vi "Begin.vi"(8 "error in":errorcluster) -> (0 "error out":errorcluster)   [LabVIEW 2018]
doc: "Called before other user functions, this VI is expected to open initial I/O refnums, load in file data, and do all program initialization. Notice that the <B>error out</B> terminal is simply used for data flow. Wiring it to other structures or subVIs ensures that this VI runs first."
uses:
  <vilib>/Rock Robotics/WPI/Encoder/WPI_EncoderType.ctl
  <vilib>/Rock Robotics/WPI/DriverStation/WPI_DriverStationRobotMode2.ctl
  <vilib>/Rock Robotics/WPI/Joystick/WPI_JoystickDeviceEnum.ctl
  <vilib>/Rock Robotics/SystemInterfaces/spilib/spi_bus.ctl
  <vilib>/Rock Robotics/WPI/Solenoid/WPI_SolenoidChannel.ctl
  <vilib>/Rock Robotics/SystemInterfaces/DIO/FPGA_DIOPWMChannel.ctl
  <vilib>/Rock Robotics/SystemInterfaces/DIO/FPGA_DIOChannel.ctl
  Robot Global Data.vi
  <vilib>/Rock Robotics/WPI/MotorControl/WPI_MotorControlOpen VictorSP.vi
  <vilib>/Rock Robotics/WPI/Counter/WPI_CounterDigitalInputToDigitalSource.vi
  <vilib>/Rock Robotics/WPI/Solenoid/WPI_SolenoidOpenDouble.vi
  navX-MXP Library/navX-MXP IMU.lvlib
  navX-MXP Library/SERIAL/IO/NI WPI/WPI_SerialPort_USB.ctl
  <vilib>/Rock Robotics/WPI/CAN/TalonSRX/WPI_CANTalonSRX_APIFeedbackSelect.ctl
  <vilib>/Rock Robotics/WPI/CAN/TalonSRX/WPI_CANTalonSRX_APIControlMode.ctl
  <vilib>/Rock Robotics/WPI/MotorControl/WPI_MotorControlOpen SD540.vi
  <vilib>/Rock Robotics/WPI/Gyro/WPI_GyroAnalogOpen.vi
panel:
  in  "Invert Direction":bool
  in  "Decoding Type":T1=enum."4x"
  in  "DistancePerCount":dbl=0.0184
  # "comp:\n?\nprac:\n0.026"
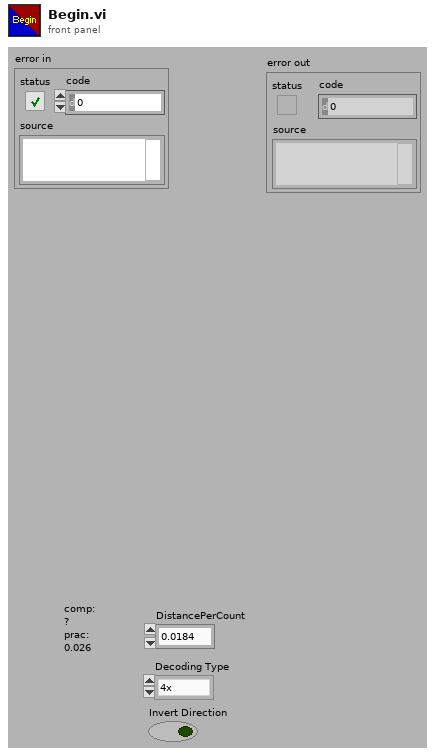
[diagram p1: front panel]
types:
  T1 = typedef "WPI_EncoderType.ctl" = enum16{"1x", "2x", "4x"}
  T2 = typedef "FPGA_DIOChannel.ctl" = enum8{"DIO 0", "DIO 1", "DIO 2", "DIO 3", "DIO 4", "DIO 5", "DIO 6", "DIO 7", "DIO 8", "DIO 9", "DIO MXP 0", "DIO MXP 1", "DIO MXP 2", "DIO MXP 3", "DIO MXP 4", "DIO MXP 5", "DIO MXP 6", "DIO MXP 7", "DIO MXP 8", "DIO MXP 9", "DIO MXP 10", "DIO MXP 11", "DIO MXP 12", "DIO MXP 13", "DIO MXP 14", "DIO MXP 15", "SPI Port CS1", "SPI Port CS2", "SPI Port CS3", "SPI Port MISO", "SPI Port MOSI", "Invalid"}
  T3 = typedef "FPGA_DIOPWMChannel.ctl" = enum8{"PWM 0", "PWM 1", "PWM 2", "PWM 3", "PWM 4", "PWM 5", "PWM 6", "PWM 7", "PWM 8", "PWM 9", "PWM MXP 0", "PWM MXP 1", "PWM MXP 2", "PWM MXP 3", "PWM MXP 4", "PWM MXP 5", "PWM MXP 6", "PWM MXP 7", "PWM MXP 8", "PWM MXP 9", "Invalid"}
  T4 = typedef "WPI_SolenoidChannel.ctl" = enum8{"Solenoid 0", "Solenoid 1", "Solenoid 2", "Solenoid 3", "Solenoid 4", "Solenoid 5", "Solenoid 6", "Solenoid 7", "Invalid"}
  T5 = typedef "spi_bus.ctl" = enum16{"SPI On-Board, CS0", "SPI On-Board, CS1", "SPI On-Board, CS2", "SPI On-Board, CS3", "SPI MXP", "Invalid"}
  T6 = typedef "WPI_JoystickDeviceEnum.ctl" = enum16{"USB 0", "USB 1", "USB 2", "USB 3", "USB 4", "USB 5"}
  T7 = typedef "WPI_DriverStationRobotMode2.ctl" = enum16{"Autonomous Disabled", "Autonomous Enabled", "Teleop Disabled", "Teleop Enabled", "Disconnected", "Finish", "Test Disabled", "Test Enabled", "Emergency Stopped"}
  T8 = typedef "WPI_DigitalInputDevRef.ctl" = cluster{"DevStatus":errorcluster, "DIO Channel":T2}
  T9 = typedef "FPGA_CounterEncoderSourceConvertionLVSourceType.ctl" = cluster{"DevStatus":errorcluster, "AnalogTriggerMode?":bool, "DigitalMode":cluster{"DIO Channel":T10}, "AnalogTriggerMode":cluster{"AnalogTriggerIndex":T11, "OutputType":T12}}
  T10 = typedef "FPGA_DIODigitalSourceChannel.ctl" = enum8{"DIO 0", "DIO 1", "DIO 2", "DIO 3", "DIO 4", "DIO 5", "DIO 6", "DIO 7", "DIO 8", "DIO 9", "DIO MXP 0", "DIO MXP 1", "DIO MXP 2", "DIO MXP 3", "DIO MXP 4", "DIO MXP 5", "DIO MXP 6", "DIO MXP 7", "DIO MXP 8", "DIO MXP 9", "DIO MXP 10", "DIO MXP 11", "DIO MXP 12", "DIO MXP 13", "DIO MXP 14", "DIO MXP 15", "SPI Port CS1", "SPI Port CS2", "SPI Port CS3", "SPI Port MISO", "SPI Port MOSI", "Disabled"}
  T11 = typedef "FPGA_AnalogTriggerIndex.ctl" = enum8{"Trig 0", "Trig 1", "Trig 2", "Trig 3", "Trig 4", "Trig 5", "Trig 6", "Trig 7", "Invalid"}
  T12 = typedef "FPGA_AnalogTriggerOutType.ctl" = enum16{"InWindow", "TriggerState", "Rising", "Falling"}
  T13 = typedef "WPI_EncoderDevRef.ctl" = cluster{"DevStatus":errorcluster, "EncoderIndex":T14, "CounterIndex":T15, "DistancePerCount":dbl, "Decoding Type":T1}
  T14 = typedef "FPGA_EncoderIdx.ctl" = enum8{"Enc 0", "Enc 1", "Enc 2", "Enc 3", "Enc 4", "Enc 5", "Enc 6", "Enc 7", "Invalid"}
  T15 = typedef "FPGA_CounterCtrSystemIndex.ctl" = enum8{"Ctr 0", "Ctr 1", "Ctr 2", "Ctr 3", "Ctr 4", "Ctr 5", "Ctr 6", "Ctr 7", "Invalid"}
  T16 = typedef "WPI_GyroDevRef.ctl" = cluster{"DevStatus":errorcluster, "Analog Channel":T17, "Gain (VoltsPerDegree/Second)":dbl, "Gyro Type":enum16{"Analog", "XRS450"}, "Handle":i32, "SPI Bus":T5, "Device Found":bool, "Sample Rate":dbl, "Calibrate On Open":bool, "Offset":dbl}
  T17 = typedef "FPGA_AIChannel.ctl" = enum8{"AI 0", "AI 1", "AI 2", "AI 3", "AI MXP 0", "AI MXP 1", "AI MXP 2", "AI MXP 3", "Invalid"}
  T18 = typedef "WPI_MotorControlDeviceRef.ctl" = cluster{"DeviceStatus":errorcluster, "Type":T19, "PWM":cluster{"PWM Channel":T3, "DeadBand":T20}, "CAN":cluster{"Device Number":u8, "SetOutput VI Ref":variant, "GetOutput VI Ref":variant, "Enable VI Ref":variant, "Disable VI Ref":variant, "Data":variant}, "Invert":bool, "DIO PWM":cluster{"PWM \"Enable\" Channel":T3, "DIOChannel":T2, "PWM Rate":dbl}}
  T19 = typedef "WPI_MotorControlType.ctl" = enum16{"PWM", "CAN", "DIO PWM"}
  T20 = typedef "WPI_PWMDeadband.ctl" = cluster{"Name":string, "maxPositivePwm":i32, "minPositivePwm":i32, "centerPwm":i32, "maxNegativePwm":i32, "minNegativePwm":i32, "angularRange":u16}
  T21 = typedef "WPI_SolenoidDevRef.ctl" = cluster{"DevStatus":errorcluster, "Pneumatics Control Module":u8, "Forward Solenoid Channel":T4, "Reverse Solenoid Channel":T4}
  T22 = typedef "navX-MXP IMU.lvlib/navX SPI DevRef.ctl" = cluster{"SPIDevRef":T23, "Board Information":T24, "Status":T25, "Offsets":cluster{"Yaw":dbl, "Quat W":dbl, "Quat X":dbl, "Quat Y":dbl, "Quat Z":dbl}, "Update Rate (4Hz-60Hz)":u8, "refnum name":string, "error":errorcluster}
  T23 = typedef "WPI_SPIDevRef.ctl" = cluster{"DevStatus":errorcluster, "Handle":i32, "SPI Bus":T5}
  T24 = typedef "navX-MXP IMU.lvlib/navX Board Information.ctl" = cluster{"WhoAmI (50 | 0x32)":u8, "Board Revision":u8, "Firmware Major Version":u8, "Firmware Minor Version":u8}
  T25 = typedef "navX-MXP IMU.lvlib/navX Status Data.ctl" = cluster{"Update Rate Hz":u8, "Accelerometer Full-Scale Range":u8, "Gyro Full-Scale Range":u16, "NAVX_OP_STATUS":T26, "NAVX_CAL_STATUS":T27, "NAVX_SELFTEST_STATUS":u8, "NAVX_SENSOR_STATUS":T28}
  T26 = typedef "navX-MXP IMU.lvlib/navX NAVX_OP_STATUS.ctl" = u8
  T27 = typedef "navX-MXP IMU.lvlib/navX NAVX_CAL_STATUS.ctl" = u8
  T28 = typedef "navX-MXP IMU.lvlib/navX NAVX_SENSOR_STATUS.ctl" = cluster{"MOVING":bool, "YAW_STABLE":bool, "MAG_DISTURBANCE":bool, "ALTITUDE_VALID":bool, "SEALEVEL_PRESS_SET":bool, "FUSED_HEADING_VALID":bool}
  T29 = typedef "WPI_JoystickDevRef.ctl" = cluster{"Device":T6}
  T30 = typedef "WPI_CANTalonSRX_APIControlMode.ctl" = enum8{"Percent VBus", "Speed", "Position", "Slave", "Unchanged / Invalid"}
  T31 = typedef "WPI_CANTalonSRX_APIFeedbackSelect.ctl" = enum16{"Digital Quadrature Encoder", "Analog Potentiometer", "Analog Encoder"}
  T32 = typedef "navX-MXP IMU.lvlib/WPI_SerialPort_USB.ctl" = enum16{"Onboard RS-232", "MXP TTL", "USB"}
  T33 = typedef "navX-MXP IMU.lvlib/navX Serial DevRef.ctl" = cluster{"SerialPortRef":T34, "Board Information":T24, "Status":T25, "Offsets":cluster{"Yaw":dbl, "Quat W":dbl, "Quat X":dbl, "Quat Y":dbl, "Quat Z":dbl}, "Update Rate (4Hz-60Hz)":u8, "Nav6Mode (YPR)":T35, "refnum name":string, "error":errorcluster}
  T34 = typedef "WPI_SerialPortRef.ctl" = cluster{"DevStatus":errorcluster, "Serial Port Name":refnum<visa-resource-name>}
  T35 = typedef "navX-MXP IMU.lvlib/navX Serial Mode.ctl" = enum16{"YPR", "Gyro", "Quaternion"}
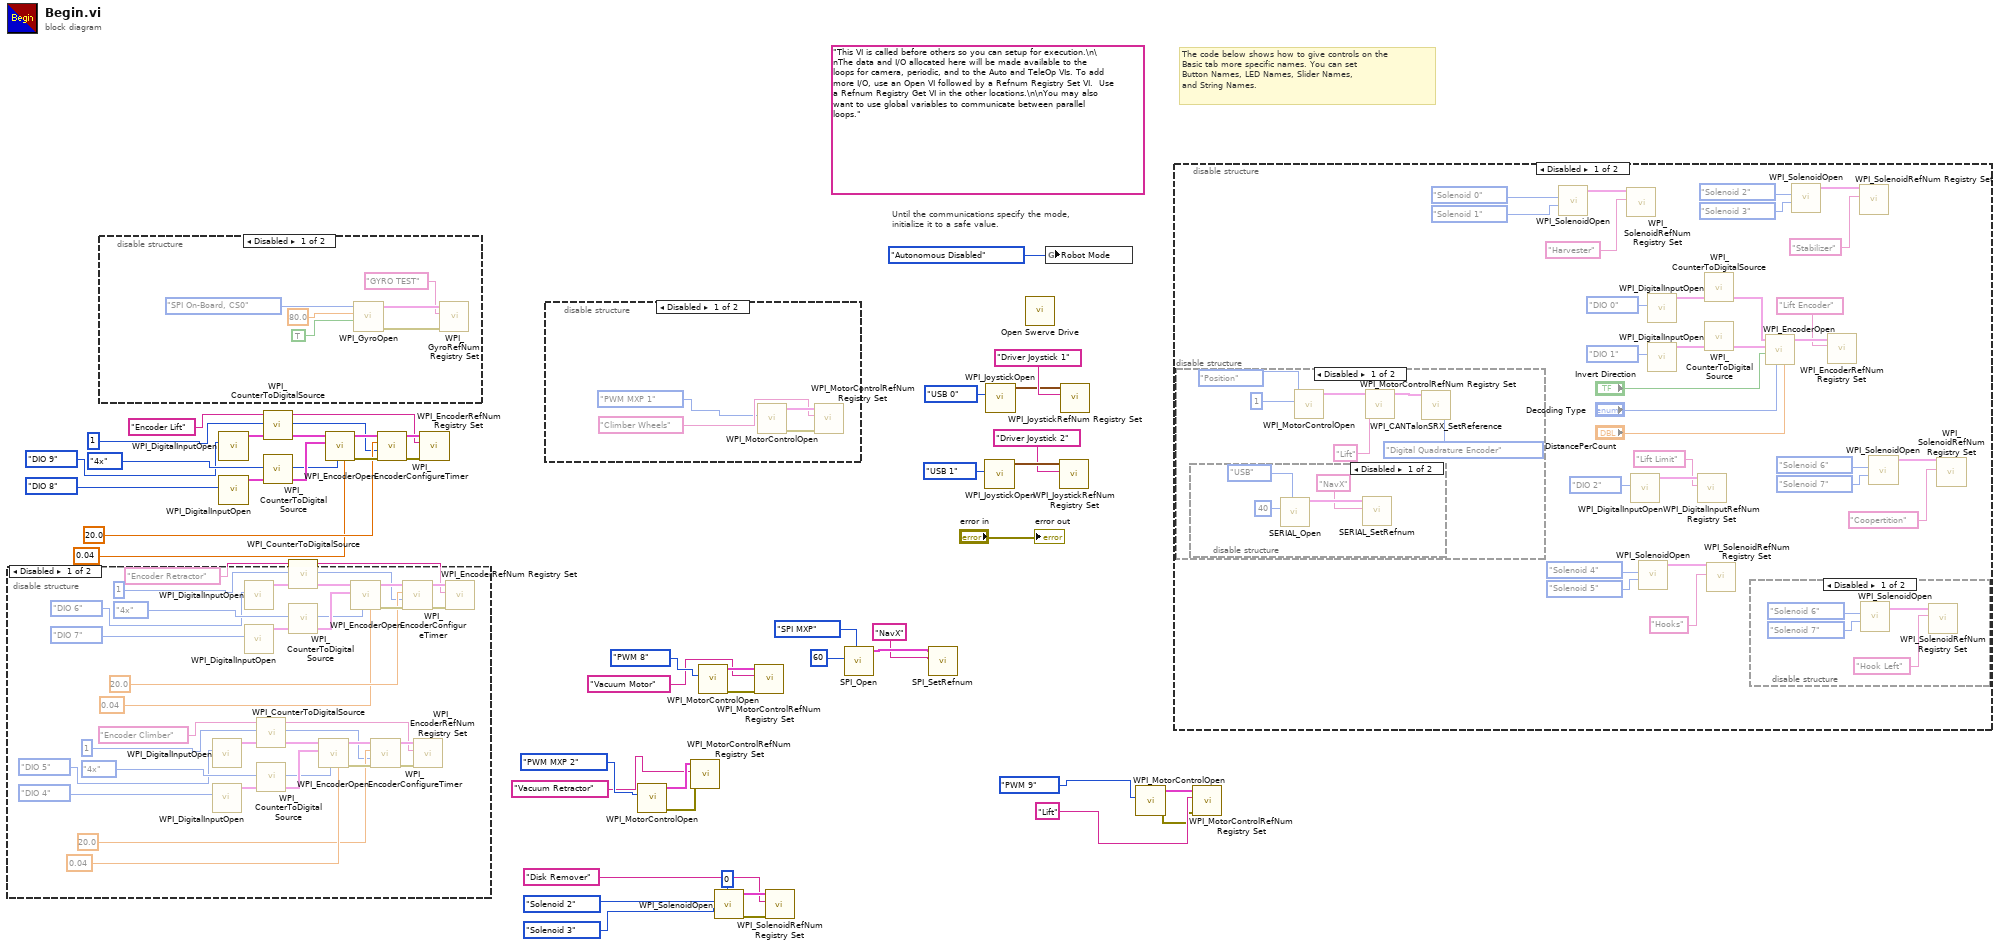
[diagram p0: block diagram]
diagram:
  (unwired) "This VI is called before others so you can setup for execution.\n\nThe data and I/O allocated here will be made available to the loops for camera, periodic, and to the Auto and TeleOp VIs. To add more I/O, use an Open VI followed by a Refnum Registry Set VI.  Use a Refnum Registry Get VI in the other locations.\n\nYou may also want to use global variables to communicate between parallel loops."
  # "The code below shows how to give controls on the\nBasic tab more specific names. You can set\nButton Names, LED Names, Slider Names,\nand String Names."
  # "Until the communications specify the mode,\ninitialize it to a safe value."
  n1 = disable-structure shown="Disabled" {
    frame Disabled {
      n2 = call <vilib>:"WPI_DigitalInputOpen.vi"("DIO Channel"=FPGA_DIOChannel."DIO 5") -> ("DigitalInputDevRef"=w73:T8)  [unwired: 1 in, 9 out]
      n3 = call <vilib>:"WPI_DigitalInputOpen.vi"("DIO Channel"=FPGA_DIOChannel."DIO 4" ("DIO Channel 2")) -> ("DigitalInputDevRef"=w74:T8)  [unwired: 1 in, 9 out]
      n4 = call <vilib>:"WPI_DigitalInputOpen.vi"("DIO Channel"=FPGA_DIOChannel."DIO 6") -> ("DigitalInputDevRef"=w58:T8)  [unwired: 1 in, 9 out]
      n5 = call <vilib>:"WPI_DigitalInputOpen.vi"("DIO Channel"=FPGA_DIOChannel."DIO 7" ("DIO Channel 2")) -> ("DigitalInputDevRef"=w59:T8)  [unwired: 1 in, 9 out]
      n6 = call-poly <vilib>:"WPI_CounterToDigitalSource.vi"("DigitalInputDevRef"=w73) -> ("Digital Source"=w72:T9)  [unwired: 6 out]
      n7 = call-poly <vilib>:"WPI_CounterToDigitalSource.vi"("DigitalInputDevRef"=w74) -> ("Digital Source"=w75:T9)  [unwired: 6 out]
      n8 = call-poly <vilib>:"WPI_CounterToDigitalSource.vi"("DigitalInputDevRef"=w58) -> ("Digital Source"=w57:T9)  [unwired: 6 out]
      n9 = call-poly <vilib>:"WPI_CounterToDigitalSource.vi"("DigitalInputDevRef"=w59) -> ("Digital Source"=w60:T9)  [unwired: 6 out]
      n10 = call <vilib>:"WPI_EncoderOpen.vi"("DistancePerCount"=0.04 ("DistancePerCount 2"), "Decoding Type"=WPI_EncoderType."4x" ("Decoding Type 2"), "BSource"=w75, "ASource"=w72) -> ("error out"=w69:errorcluster, "EncoderDevRef"=w71:T13)  [unwired: 4 in, 2 out]
      n11 = call <vilib>:"WPI_EncoderOpen.vi"("DistancePerCount"=0.04 ("DistancePerCount 2"), "Decoding Type"=WPI_EncoderType."4x" ("Decoding Type 2"), "BSource"=w60, "ASource"=w57) -> ("error out"=w54:errorcluster, "EncoderDevRef"=w56:T13)  [unwired: 4 in, 2 out]
      n12 = call <vilib>:"WPI_EncoderConfigureTimer.vi"("error in (no error)"=w69, "Number Samples to Average"=u8 1, "Minimum Rate"=20.0, "EncoderDevRef"=w71) -> ("error out"=w68:errorcluster, "EncoderDevRef"=w70:T13)  [unwired: 6 in]
      n13 = call <vilib>:"WPI_EncoderConfigureTimer.vi"("error in (no error)"=w54, "Number Samples to Average"=u8 1, "Minimum Rate"=20.0, "EncoderDevRef"=w56) -> ("error out"=w53:errorcluster, "EncoderDevRef"=w55:T13)  [unwired: 6 in]
      n14 = call <vilib>:"WPI_EncoderRefNum Registry Set.vi"("error in (no error)"=w68, "refnum name"="Encoder Climber", "EncoderDevRef"=w70) -> ()  [unwired: 7 in, 2 out]
      n15 = call <vilib>:"WPI_EncoderRefNum Registry Set.vi"("error in (no error)"=w53, "refnum name"="Encoder Retractor", "EncoderDevRef"=w55) -> ()  [unwired: 7 in, 2 out]
    }
    frame Enabled {
    }
  }
  n16 = disable-structure shown="Disabled" {
    frame Disabled {
      n17 = call-poly <vilib>:"WPI_GyroOpen.vi"("Calibrate On Open"=TRUE, "Analog Channel"=80.0 ("Sample Rate (Hz)"), 11:spi_bus."SPI On-Board, CS0" ("SPI Bus")) -> ("error out"=w80:errorcluster, "GyroDevRef"=w81:T16)  [unwired: 6 in, 1 out]
      n18 = call <vilib>:"WPI_GyroRefNum Registry Set.vi"("error in (no error)"=w80, "refnum name"="GYRO TEST", "GyroDevRef"=w81) -> ()  [unwired: 7 in, 2 out]
    }
    frame Enabled {
    }
  }
  n19 = call <vilib>:"WPI_DigitalInputOpen.vi"("DIO Channel"=FPGA_DIOChannel."DIO 9") -> ("DigitalInputDevRef"=w19:T8)  [unwired: 1 in, 9 out]
  n20 = call <vilib>:"WPI_DigitalInputOpen.vi"("DIO Channel"=FPGA_DIOChannel."DIO 8" ("DIO Channel 2")) -> ("DigitalInputDevRef"=w20:T8)  [unwired: 1 in, 9 out]
  n21 = call-poly <vilib>:"WPI_CounterToDigitalSource.vi"("DigitalInputDevRef"=w19) -> ("Digital Source"=w18:T9)  [unwired: 6 out]
  n22 = call-poly <vilib>:"WPI_CounterToDigitalSource.vi"("DigitalInputDevRef"=w20) -> ("Digital Source"=w21:T9)  [unwired: 6 out]
  n23 = call <vilib>:"WPI_EncoderOpen.vi"("DistancePerCount"=0.04 ("DistancePerCount 2"), "Decoding Type"=WPI_EncoderType."4x" ("Decoding Type 2"), "BSource"=w21, "ASource"=w18) -> ("error out"=w15:errorcluster, "EncoderDevRef"=w17:T13)  [unwired: 4 in, 2 out]
  n24 = call <vilib>:"WPI_EncoderConfigureTimer.vi"("error in (no error)"=w15, "Number Samples to Average"=u8 1, "Minimum Rate"=20.0, "EncoderDevRef"=w17) -> ("error out"=w14:errorcluster, "EncoderDevRef"=w16:T13)  [unwired: 6 in]
  n25 = call <vilib>:"WPI_EncoderRefNum Registry Set.vi"("error in (no error)"=w14, "refnum name"="Encoder Lift", "EncoderDevRef"=w16) -> ()  [unwired: 7 in, 2 out]
  n26 = disable-structure shown="Disabled" {
    frame Disabled {
      n27 = call-poly <vilib>:"WPI_MotorControlOpen.vi"("PWM Channel"=FPGA_DIOPWMChannel."PWM MXP 1") -> ("error out"=w85:errorcluster, "MotorControlDeviceRef"=w84:T18)  [unwired: 9 in]
      n28 = call <vilib>:"WPI_MotorControlRefNum Registry Set.vi"("error in (no error)"=w85, "refnum name"="Climber Wheels", "MotorControlDevRef"=w84) -> ()  [unwired: 7 in, 2 out]
    }
    frame Enabled {
    }
  }
  n29 = call-poly <vilib>:"WPI_MotorControlOpen.vi"("PWM Channel"=FPGA_DIOPWMChannel."PWM MXP 2") -> ("error out"=w28:errorcluster, "MotorControlDeviceRef"=w29:T18)  [unwired: 9 in]
  n30 = call <vilib>:"WPI_MotorControlRefNum Registry Set.vi"("error in (no error)"=w28, "refnum name"="Vacuum Retractor", "MotorControlDevRef"=w29) -> ()  [unwired: 7 in, 2 out]
  n31 = call-poly <vilib>:"WPI_MotorControlOpen.vi"("PWM Channel"=FPGA_DIOPWMChannel."PWM 8") -> ("error out"=w30:errorcluster, "MotorControlDeviceRef"=w33:T18)  [unwired: 9 in]
  n32 = call-poly <vilib>:"WPI_SolenoidOpen.vi"("Reverse Solenoid Channel"=WPI_SolenoidChannel."Solenoid 3", "Forward Solenoid Channel"=WPI_SolenoidChannel."Solenoid 2" ("Solenoid Channel"), "Pneumatics Control Module (0)"=u8 0) -> ("error out"=w5:errorcluster, "SolenoidDevRef"=w6:T21)  [unwired: 7 in]
  n33 = call <vilib>:"WPI_MotorControlRefNum Registry Set.vi"("error in (no error)"=w30, "refnum name"="Vacuum Motor", "MotorControlDevRef"=w33) -> ()  [unwired: 7 in, 2 out]
  n34 = call <vilib>:"WPI_SolenoidRefNum Registry Set.vi"("error in (no error)"=w5, "refnum name"="Disk Remover", "SolenoidDevRef"=w6) -> ()  [unwired: 7 in, 2 out]
  n35 = call "SPI_Open.vi"("SPI Bus (SPI MXP)"=spi_bus."SPI MXP", "Update Rate (4Hz-60Hz)"=u8 60) -> ("navX DevRef"=w36:T22)  [unwired: 7 in, 2 out]
  n36 = call "SPI_SetRefnum.vi"("refnum name"="NavX", "navX DevRef"=w36) -> ()  [unwired: 8 in, 2 out]
  n37 = call <vilib>:"WPI_JoystickOpen.vi"("JoystickDevice"=WPI_JoystickDeviceEnum."USB 1") -> ("JoystickDevRef"=w39:T29)  [unwired: 10 in]
  n38 = call <vilib>:"WPI_JoystickOpen.vi"("JoystickDevice"=WPI_JoystickDeviceEnum."USB 0") -> ("JoystickDevRef"=w43:T29)  [unwired: 10 in]
  n39 = call "Open Swerve Drive.vi"() -> ()  [unwired: 12 in]
  n40 = global write "Robot Global Data.vi" "Robot Mode"(WPI_DriverStationRobotMode2."Autonomous Disabled" ("Robot Mode")) -> ()
  n41 = call <vilib>:"WPI_JoystickRefNum Registry Set.vi"("refnum name"="Driver Joystick 2", "JoystickDevRef"=w39) -> ()  [unwired: 8 in, 2 out]
  n42 = call <vilib>:"WPI_JoystickRefNum Registry Set.vi"("refnum name"="Driver Joystick 1", "JoystickDevRef"=w43) -> ()  [unwired: 8 in, 2 out]
  n43 = call-poly <vilib>:"WPI_MotorControlOpen.vi"("PWM Channel"=FPGA_DIOPWMChannel."PWM 9") -> ("error out"=w22:errorcluster, "MotorControlDeviceRef"=w23:T18)  [unwired: 9 in]
  n44 = disable-structure shown="Disabled" {
    frame Disabled {
      n45 = disable-structure shown="Disabled" {
        frame Disabled {
          n46 = disable-structure shown="Disabled" {
            frame Disabled {
              n47 = call "SERIAL_Open.vi"("Serial Port (MXP)"=WPI_SerialPort_USB."USB", "Update Rate (4Hz-60Hz)"=u8 40) -> ("navX Ref"=w124:T33)  [unwired: 7 in, 2 out]
              n48 = call "SERIAL_SetRefnum.vi"("refnum name"="NavX", "navX DevRef"=w124) -> ()  [unwired: 8 in, 2 out]
            }
            frame Enabled {
            }
          }
          n49 = call-poly <vilib>:"WPI_MotorControlOpen.vi"("PWM Channel"=u8 1 ("Device Number"), 11:WPI_CANTalonSRX_APIControlMode."Position" ("Control Mode")) -> ("MotorControlDeviceRef"=w120:T18)  [unwired: 8 in, 1 out]
          n50 = call <vilib>:"WPI_MotorControlRefNum Registry Set.vi"("refnum name"="Lift", "MotorControlDevRef"=w120) -> ("MotorControlDevRef"=w118:T18)  [unwired: 8 in, 1 out]
          n51 = call <vilib>:"WPI_CANTalonSRX_SetReference.vi"("Feedback Reference"=WPI_CANTalonSRX_APIFeedbackSelect."Digital Quadrature Encoder", "CAN Talon SRX Ref"=w118) -> ()  [unwired: 8 in, 2 out]
        }
        frame Enabled {
        }
      }
      n52 = call-poly <vilib>:"WPI_SolenoidOpen.vi"("Reverse Solenoid Channel"=WPI_SolenoidChannel."Solenoid 1", "Forward Solenoid Channel"=WPI_SolenoidChannel."Solenoid 0" ("Solenoid Channel")) -> ("SolenoidDevRef"=w100:T21)  [unwired: 8 in, 1 out]
      n53 = call <vilib>:"WPI_SolenoidRefNum Registry Set.vi"("refnum name"="Harvester", "SolenoidDevRef"=w100) -> ()  [unwired: 8 in, 2 out]
      n54 = call <vilib>:"WPI_DigitalInputOpen.vi"("DIO Channel"=FPGA_DIOChannel."DIO 2") -> ("DigitalInputDevRef"=w103:T8)  [unwired: 1 in, 9 out]
      n55 = call-poly <vilib>:"WPI_SolenoidOpen.vi"("Reverse Solenoid Channel"=WPI_SolenoidChannel."Solenoid 5", "Forward Solenoid Channel"=WPI_SolenoidChannel."Solenoid 4" ("Solenoid Channel")) -> ("SolenoidDevRef"=w92:T21)  [unwired: 8 in, 1 out]
      n56 = call <vilib>:"WPI_DigitalInputOpen.vi"("DIO Channel"=FPGA_DIOChannel."DIO 0") -> ("DigitalInputDevRef"=w113:T8)  [unwired: 1 in, 9 out]
      n57 = call <vilib>:"WPI_DigitalInputOpen.vi"("DIO Channel"=FPGA_DIOChannel."DIO 1") -> ("DigitalInputDevRef"=w114:T8)  [unwired: 1 in, 9 out]
      n58 = call <vilib>:"WPI_DigitalInputRefNum Registry Set.vi"("refnum name"="Lift Limit", "DigitalInputDevRef"=w103) -> ()  [unwired: 8 in, 2 out]
      n59 = call-poly <vilib>:"WPI_CounterToDigitalSource.vi"("DigitalInputDevRef"=w113) -> ("Digital Source"=w112:T9)  [unwired: 6 out]
      n60 = call-poly <vilib>:"WPI_CounterToDigitalSource.vi"("DigitalInputDevRef"=w114) -> ("Digital Source"=w115:T9)  [unwired: 6 out]
      n61 = call <vilib>:"WPI_SolenoidRefNum Registry Set.vi"("refnum name"="Hooks", "SolenoidDevRef"=w92) -> ()  [unwired: 8 in, 2 out]
      n62 = disable-structure shown="Disabled" {
        frame Disabled {
          n63 = call-poly <vilib>:"WPI_SolenoidOpen.vi"("Reverse Solenoid Channel"=WPI_SolenoidChannel."Solenoid 7", "Forward Solenoid Channel"=WPI_SolenoidChannel."Solenoid 6" ("Solenoid Channel")) -> ("SolenoidDevRef"=w126:T21)  [unwired: 8 in, 1 out]
          n64 = call <vilib>:"WPI_SolenoidRefNum Registry Set.vi"("refnum name"="Hook Left", "SolenoidDevRef"=w126) -> ()  [unwired: 8 in, 2 out]
        }
        frame Enabled {
        }
      }
      n65 = call <vilib>:"WPI_EncoderOpen.vi"("DistancePerCount"="DistancePerCount", "Decoding Type"="Decoding Type", "Invert Direction (False)"="Invert Direction", "BSource"=w115, "ASource"=w112) -> ("EncoderDevRef"=w106:T13)  [unwired: 3 in, 3 out]
      n66 = call-poly <vilib>:"WPI_SolenoidOpen.vi"("Reverse Solenoid Channel"=WPI_SolenoidChannel."Solenoid 3", "Forward Solenoid Channel"=WPI_SolenoidChannel."Solenoid 2" ("Solenoid Channel")) -> ("SolenoidDevRef"=w95:T21)  [unwired: 8 in, 1 out]
      n67 = call <vilib>:"WPI_EncoderRefNum Registry Set.vi"("refnum name"="Lift Encoder", "EncoderDevRef"=w106) -> ()  [unwired: 8 in, 2 out]
      n68 = call <vilib>:"WPI_SolenoidRefNum Registry Set.vi"("refnum name"="Stabilizer", "SolenoidDevRef"=w95) -> ()  [unwired: 8 in, 2 out]
      n69 = call-poly <vilib>:"WPI_SolenoidOpen.vi"("Reverse Solenoid Channel"=WPI_SolenoidChannel."Solenoid 7", "Forward Solenoid Channel"=WPI_SolenoidChannel."Solenoid 6" ("Solenoid Channel")) -> ("SolenoidDevRef"=w88:T21)  [unwired: 8 in, 1 out]
      n70 = call <vilib>:"WPI_SolenoidRefNum Registry Set.vi"("refnum name"="Coopertition", "SolenoidDevRef"=w88) -> ()  [unwired: 8 in, 2 out]
    }
    frame Enabled {
    }
  }
  n71 = call <vilib>:"WPI_MotorControlRefNum Registry Set.vi"("error in (no error)"=w22, "refnum name"="Lift", "MotorControlDevRef"=w23) -> ()  [unwired: 7 in, 2 out]
  "error out" <- "error in"
